vi "Enque Image (BG) (SubVI).vi"(8 "Enque":bool, 10 "Image Array":u64[](array[numeric]), 11 "BG Image REF":refnum<queue>) -> ()   [LabVIEW 2020]
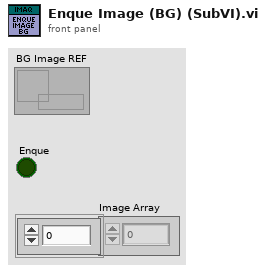
[diagram p1: front panel]
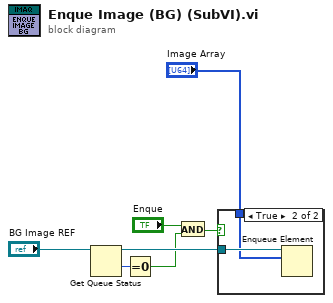
[diagram p0: block diagram]
diagram:
  n1 = Get Queue Status(queue="BG Image REF") -> (queue out=w5:refnum<queue>, # elements in queue=w2:i32)  [unwired: 2 in, 6 out]
  n2 = Equal To 0?(x=w2) -> (x = 0?=w3:bool)
  n3 = And(x="Enque", y=w3) -> (x .and. y?=w4:bool)
  n4 = case shown="True" w4 {
    tunnel: w5 -> [_ w9]
    tunnel: "Image Array" -> [_ w8]
    frame False {
    }
    frame True {
      n5 = Enqueue Element(queue=w9, element=w8) -> ()  [unwired: 2 in, 3 out]
    }
  }
